vi "WavaFrequencyMeasurement2.vi"() -> ()   [LabVIEW 2019]
uses:
  <vilib>/Platform/TimedLoop/XDataNode/timing_clust.ctl
  <vilib>/Platform/TimedLoop/XDataNode/nitl_modes.ctl
  <vilib>/Platform/TimedLoop/XDataNode/wakeup.ctl
  <vilib>/rvi/Emulation/niFpgaSctlEmulationGetInTimedLoop.vi
  <vilib>/rvi/Emulation/niFpgaEmulationReportErrorSimple.vi
  <vilib>/rvi/Emulation/niFpgaGetClockAttributes.vi
  <vilib>/rvi/Emulation/niFpgaCriticalErrorInLSC.vi
  <vilib>/rvi/eio/common/nirviEmuTemplateMethod_errors.vi
  <vilib>/Platform/TimedLoop/XDataNode/XDataNode.xnode
  <vilib>/eio/EIONode/EIONode.xnode
  <vilib>/Platform/TimedLoop/XDataNode/XDNodeRunTimeDep.lvlib
panel:
  out "波形图表 2":cluster{u32, u32}(graph)
  out "时钟信号个数 2":u32
  out "被测信号个数 2":u32
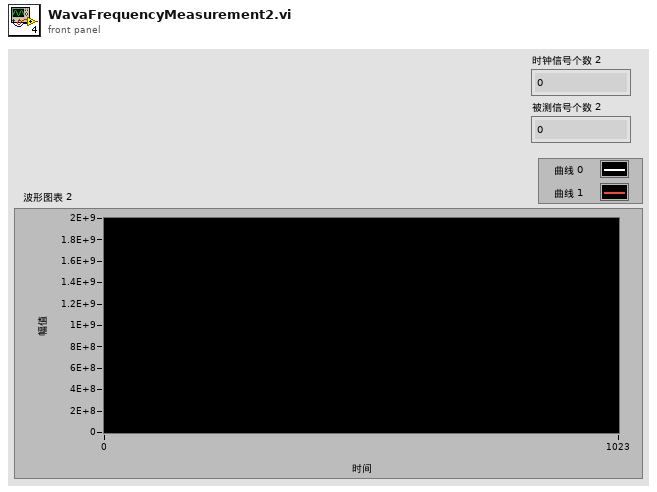
[diagram p1: front panel]
types:
  T1 = typedef "XDNodeRunTimeDep.lvlib/timing_clust.ctl" = cluster{"Expected End [f-1]":u64, "Actual End [f-1]":u64, "Finished Late? [f-1]":bool, "Expected End [i-1]":u64, "Actual End [i-1]":u64, "Finished Late? [i-1]":bool, "Expected Start [i]":u64, "Actual Start [i]":u64, "Expected Start [f]":u64, "Actual Start [f]":u64, "Source Name":string, "Structure Name":string, "Period":i64, "Deadline":i64, "Offset":i64, "Start":i64, "Priority":i32, "Timeout":i32, "Mode":T2, "Wakeup Reason":T3, "Error":errorcluster, "Source Type":string, "Secondary Source Type":string, "Global End Time":u64, "Global Start Time":u64, "Frame Duration":u64, "Iteration Duration":u64, "Assigned CPU":i32, "I/O Scan Engine Mode":u32}
  T2 = typedef "XDNodeRunTimeDep.lvlib/nitl_modes.ctl" = enum32{"No Change", "Process missed periods, maintain original phase", "Discard missed periods, maintain original phase", "Process missed periods, ignore original phase", "Discard missed periods, ignore original phase"}
  T3 = typedef "XDNodeRunTimeDep.lvlib/wakeup.ctl" = enum32{"Normal", "Aborted", "Asynchronous wakeup", "Timing source error", "Timed loop error", "Timeout"}
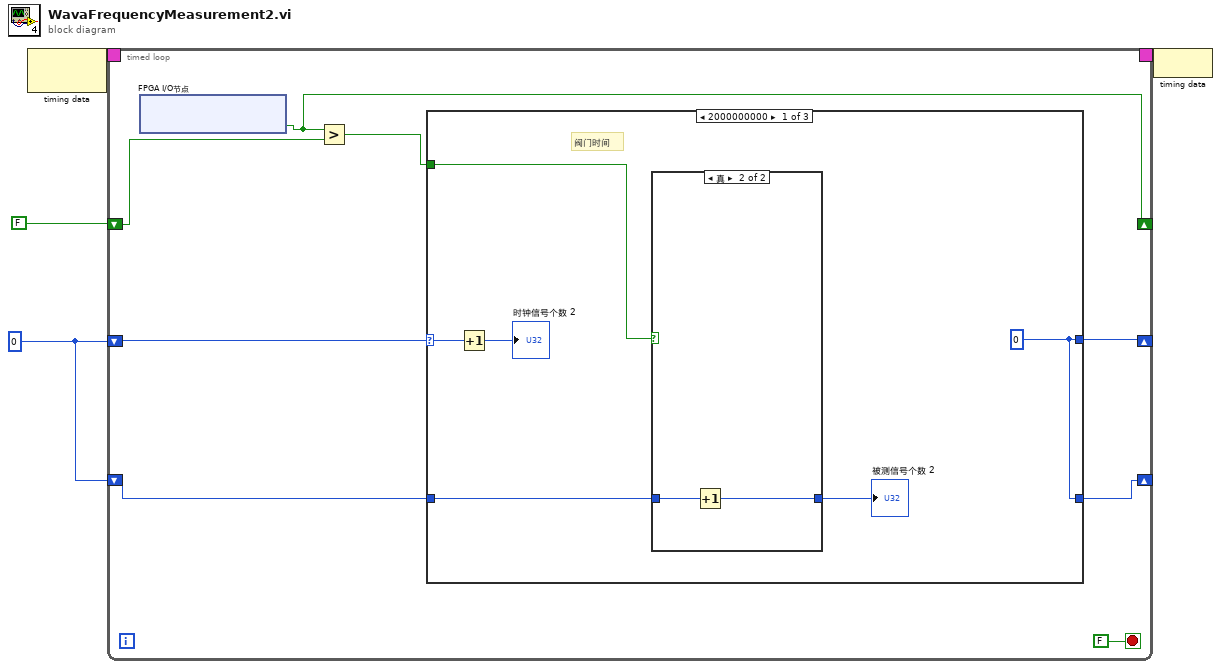
[diagram p0: block diagram]
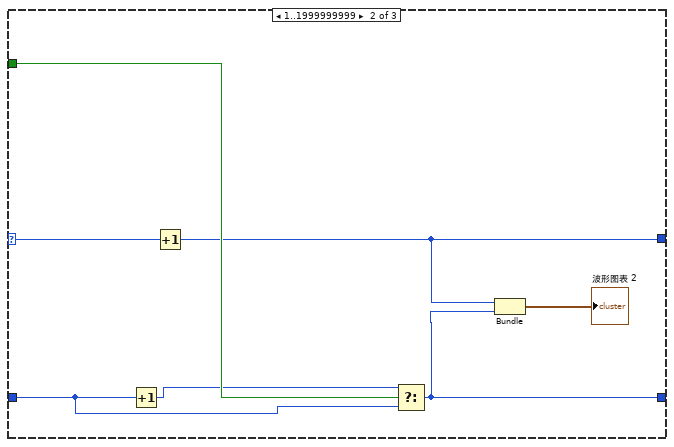
[diagram p3: hidden frame]
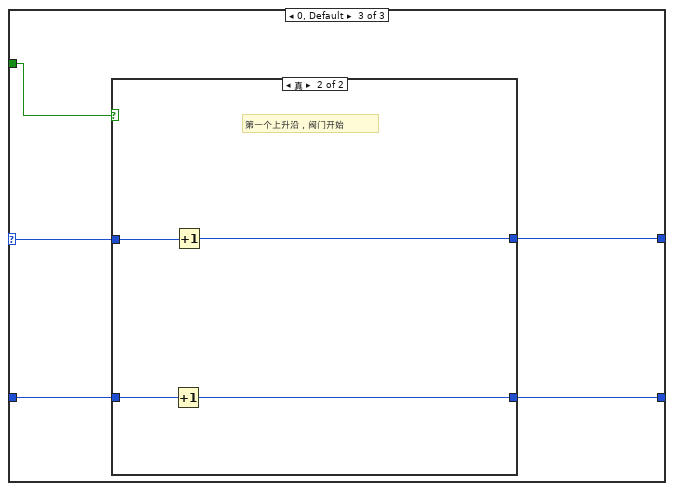
[diagram p4: hidden frame]
diagram:
  w2 = u32 0
  n1 = node-c288() -> (w4:T1)  [unwired: 1 in]
  n2 = timed-loop {
    timing: w4 -> [_]
    timing-out: [_] -> w3
    shift-right: [w11] -> _
    shift-left: FALSE -> [w12]
    shift-right: [w6] -> _
    shift-left: w2 -> [w9]
    shift-right: [w5] -> _
    shift-left: w2 -> [w8]
    stop <- FALSE stop-if-true
    n3 = xnode "FPGA I/O节点"() -> ("ConnectorB/DIO0"=w11:bool)  [unwired: 1 in, 1 out]
    n4 = Greater?(x=w11, y=w12) -> (0:w10:bool)
    n5 = case "条件结构" shown="2000000000" w9 {
      selector: w9 -> [w16 w28 w32]
      tunnel: w10 -> [w17 w26 w33]
      tunnel: w8 -> [w14 w27 w31]
      tunnel: [w18 w25 w30] -> w6
      tunnel: [w18 w23 w29] -> w5
      frame 2000000000 {
        w18 = u32 0
        # "阀门时间"
        n6 = Increment(x=w16) -> (x+1=→"时钟信号个数 2":u32)
        n7 = case shown="真" w17 {
          tunnel: w14 -> [w19 w21]
          tunnel: [w19 w20] -> w13
          frame False {
          }
          frame True {
            n8 = Increment(x=w21) -> (x+1=w20:u32)
          }
        }
        "被测信号个数 2" <- w13
      }
      frame 1..1999999999 {
        n9 = Increment(x=w27) -> (x+1=w24:u32)
        n10 = Increment(x=w28) -> (x+1=w25:u32)
        n11 = Select(t=w24, s=w26, f=w27) -> (s? t:f=w23:u32)
        n12 = Bundle(w25, w23) -> (→"波形图表 2":cluster{u32, u32})  [unwired: 1 in]
      }
      frame 0, Default {
        n13 = case shown="真" w33 {
          tunnel: w32 -> [w35 w39]
          tunnel: w31 -> [w34 w38]
          tunnel: [w35 w37] -> w30
          tunnel: [w34 w36] -> w29
          frame False {
            # "不开始"
          }
          frame True {
            # "第一个上升沿，阀门开始"
            n14 = Increment(x=w38) -> (x+1=w36:u32)
            n15 = Increment(x=w39) -> (x+1=w37:u32)
          }
        }
      }
    }
  }
  n16 = node-c288(w3) -> ()
